vi "Butterfly_extract_and_Publish_VPI_VRL - HLH - MultipleThresholds.vi"(6 "Voltages Array":dbl[](array[numeric]), 7 "ID Prefix":string, 8 "error in (no error)":errorcluster, 9 "Thresholds":dbl[](array[numeric]), 10 "Result Array In":dbl[][](array[numeric]), 11 "Semiconductor Module Context":T1) -> (0 "error out":errorcluster)   [LabVIEW 2013]
uses:
  <vilib>/NI_TestStand_SemiconductorModule/NI_TestStand_Semiconductor_Module.lvlibp/PinMap/General/SemiconductorModuleContext.ctl
  Butterfly_extract_VPI_VRL - HLH.vi
  <vilib>/NI_TestStand_SemiconductorModule/NI_TestStand_Semiconductor_Module.lvlibp/PinMap/General/Publish/PublishDataDoubleFunctionalTest.vi
  <vilib>/NI_TestStand_SemiconductorModule/NI_TestStand_Semiconductor_Module.lvlibp
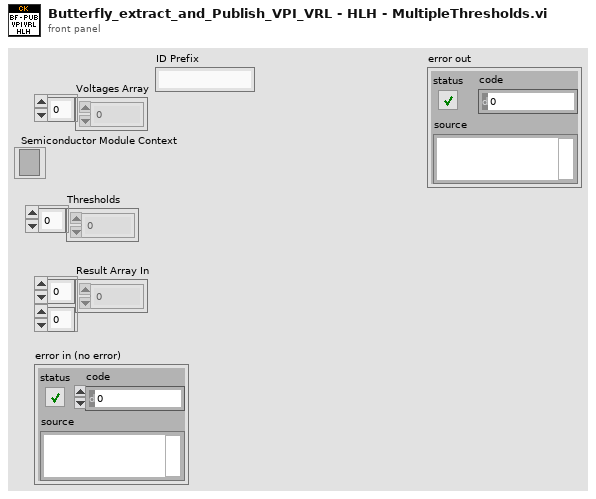
[diagram p1: front panel]
types:
  T1 = typedef "NI_TestStand_Semiconductor_Module.lvlibp/SemiconductorModuleContext.ctl" = refnum<k7>
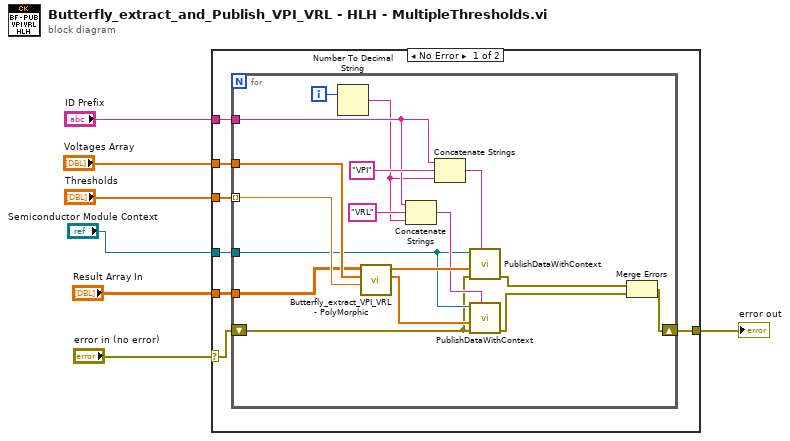
[diagram p0: block diagram]
diagram:
  n1 = case shown="No Error" "error in (no error)" {
    selector: "error in (no error)" -> [w8 w32]
    tunnel: "Thresholds" -> [w14 _]
    tunnel: "Voltages Array" -> [w13 _]
    tunnel: "Result Array In" -> [w12 _]
    tunnel: "ID Prefix" -> [w11 _]
    tunnel: "Semiconductor Module Context" -> [w10 _]
    tunnel: [w9 w32] -> w2
    frame No Error {
      n2 = for {
        tunnel: w14 -> [w29] mode=indexing
        tunnel: w13 -> [w28]
        tunnel: w12 -> [w27]
        tunnel: w11 -> [w23]
        tunnel: w10 -> [w21]
        shift-right: [w18] -> w9
        shift-left: w8 -> [w17]
        i -> [w16]
        n3 = Number To Decimal String(number=w16) -> (decimal integer string=w15:string)  [unwired: 1 in]
        n4 = call-poly "Butterfly_extract_VPI_VRL - PolyMorphic.vi"("Threshold"=w29, "Voltage Array"=w28, "Result Array In"=w27) -> ("VRLs"=w31:dbl[], "VPIs"=w30:dbl[])  [unwired: 7 in]
        n5 = Concatenate Strings(w23, "VRL" ("Published Data Id"), w15) -> (w22:string)
        n6 = Concatenate Strings(w23, "VPI" ("Published Data Id"), w15) -> (w26:string)
        n7 = call-poly <vilib>:"PublishDataWithContext.vi"("Published Data Id"=w26, "error in (no error)"=w17, "Data In"=w30, "Semiconductor Module Context"=w21) -> ("error out"=w20:errorcluster)  [unwired: 6 in, 1 out]
        n8 = call-poly <vilib>:"PublishDataWithContext.vi"("Published Data Id"=w22, "error in (no error)"=w17, "Data In"=w31, "Semiconductor Module Context"=w21) -> ("error out"=w19:errorcluster)  [unwired: 6 in, 1 out]
        n9 = Merge Errors(w20, w19) -> (w18:errorcluster)
      }
    }
    frame Error {
    }
  }
  "error out" <- w2
